vi "Tosca-Table to Schedule Params.vi"(0 "Table In":T1[](array[typedef]), 7 "Param Table":refnum<vi>) -> (4 "Table Out":T1[](array[typedef]))   [LabVIEW 2020]
uses:
  epl-vi-lib/Utility VIs/Controls/KTable/KTable.xctl
  Typedefs/Tosca-Parameter Table Element.ctl
  Typedefs/Tosca-Parameter Dimension.ctl
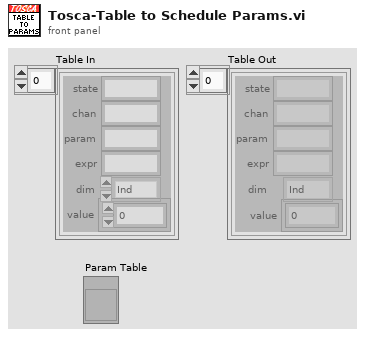
[diagram p1: front panel]
types:
  T1 = typedef "Tosca-Parameter Table Element.ctl" = cluster{"state":string, "chan":string, "param":string, "expr":string, "dim":T2, "value":dbl[]}
  T2 = typedef "Tosca-Parameter Dimension.ctl" = enum16{"Ind", "X", "Y"}
  T3 = cluster{string, string, string, "Dim":T2, string}
  T4 = cluster{string, string, string, "Dim":T2, string}[]
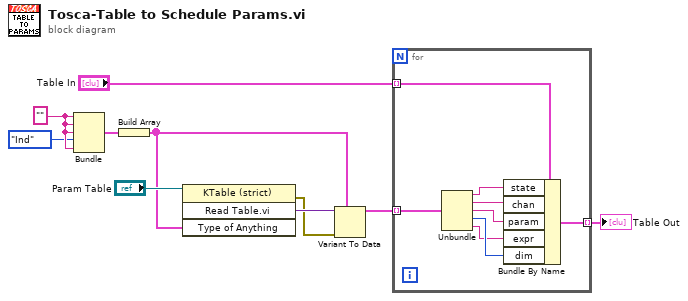
[diagram p0: block diagram]
diagram:
  w9 = ""
  n1 = Bundle(w9, w9, w9, "Dim"=Tosca-Parameter_Dimension."Ind", w9) -> (w8:T3)  [unwired: 1 in]
  n2 = Build Array(w8) -> (w5:T4)
  n3 = invoke class="KTable (strict)" method="Read Table.vi"(reference="Param Table", "Type of Anything"=w5) -> (error out=w6:errorcluster, "Read Table.vi"=w7:variant)  [unwired: 2 in, 2 out]
  n4 = Variant To Data(error in=w6, type=w5, Variant=w7) -> (data=w4:T4)  [unwired: 1 out]
  n5 = for {
    tunnel: w4 -> [w18] mode=indexing
    tunnel: [w12] -> w3 mode=indexing
    tunnel: "Table In" -> [w11] mode=indexing
    n6 = Unbundle(w18) -> (w17:string, w16:string, w15:string, "Dim"=w14:T2, w13:string)
    n7 = Bundle By Name(cluster=w11, "state"=w17, "chan"=w16, "param"=w15, "expr"=w13, "dim"=w14) -> (w12:T1)
  }
  "Table Out" <- w3
